vi "getRequirementsDoc.vi"(8 "error in (no error)":errorcluster, 11 "Path":path=path "C:/Users/rolalla/SE/Opps/2010/Harley Davidson/TestBuilder/Source/HD_TestBuilder(06152010)/Requirements Gateway 1.1/NIGEL Engine/Document/NIGEL Dynamic Test Requirements.doc") -> (0 "error out":errorcluster, 1 "Cancelled?":bool, 2 "Requirements":string[](array[string]), 3 "Req Doc Folder":path)   [LabVIEW 2011]
uses:
  Progress.vi
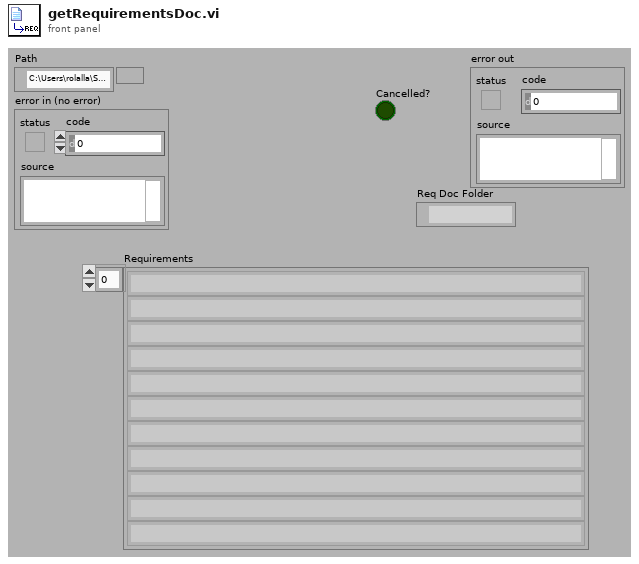
[diagram p1: front panel]
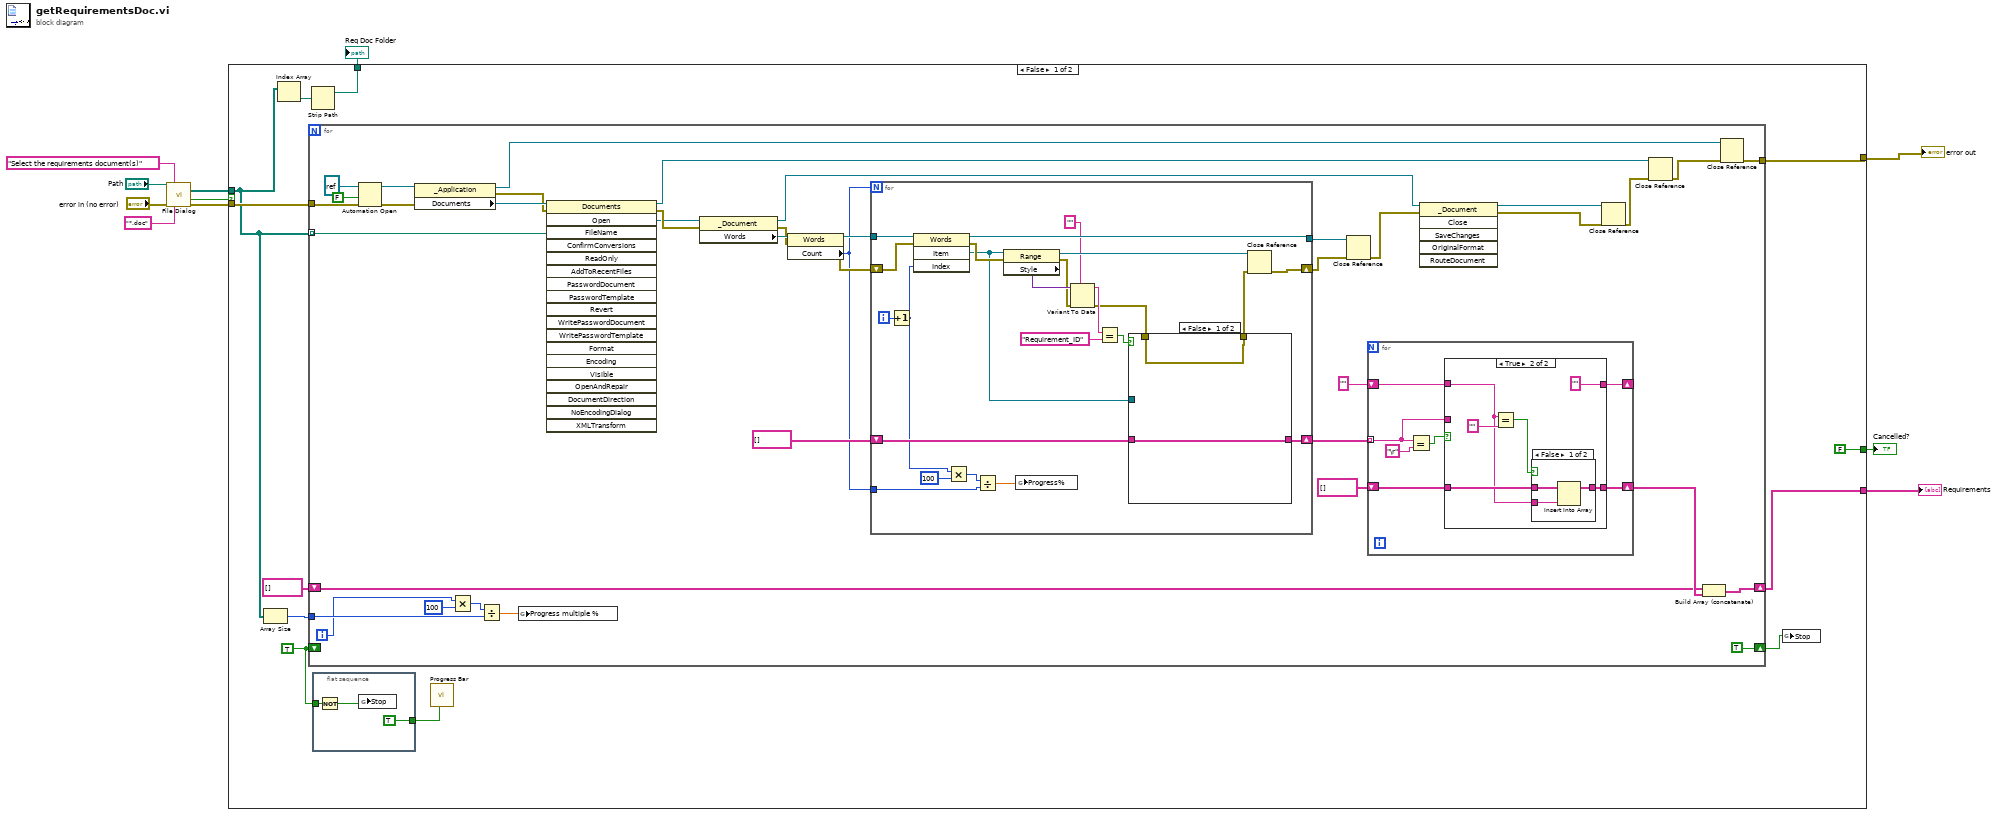
[diagram p0: block diagram]
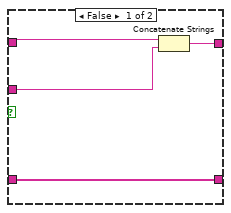
[diagram p2: hidden frame]
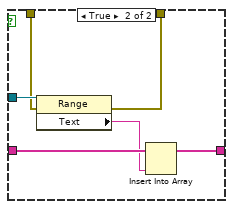
[diagram p4: hidden frame]
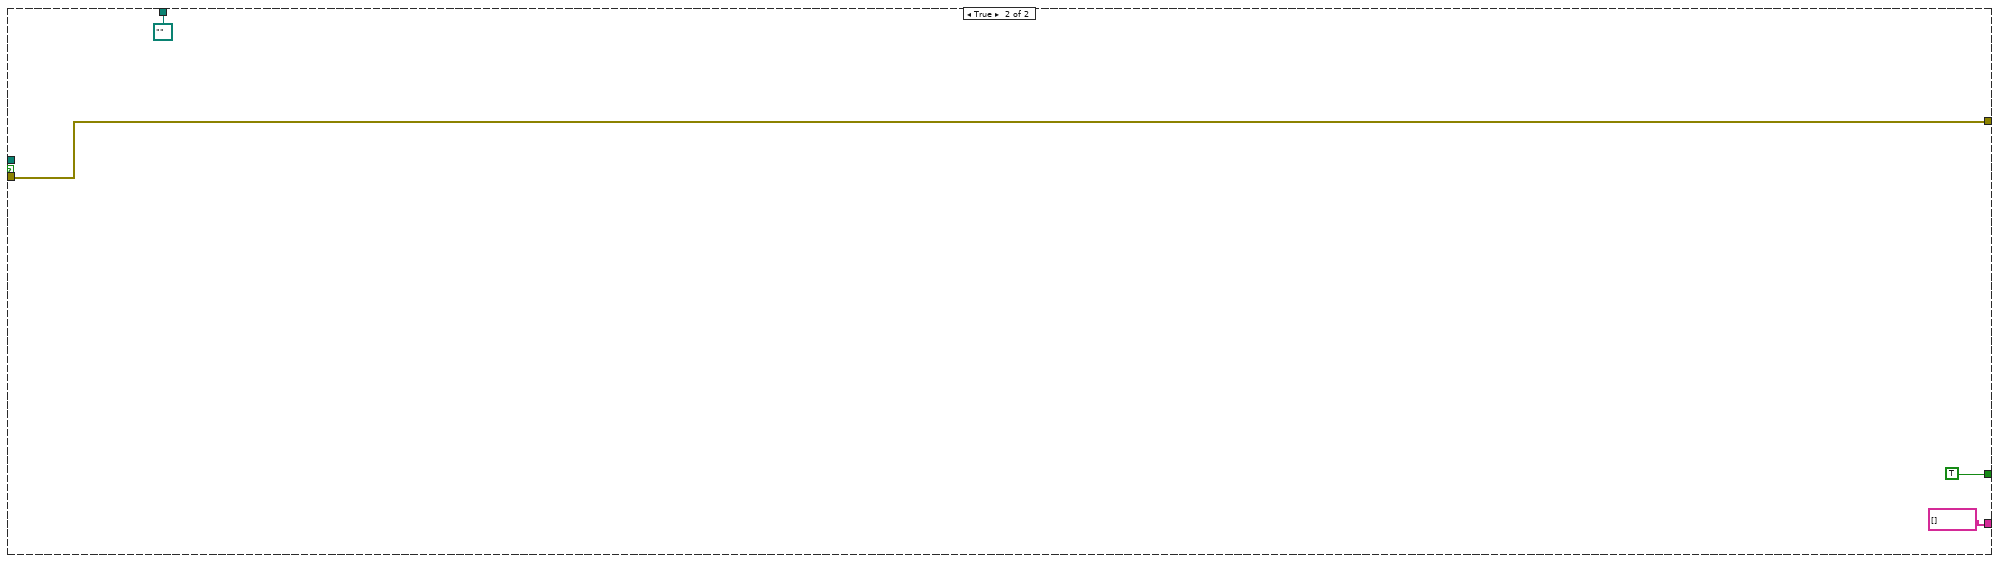
[diagram p5: hidden frame]
diagram:
  n1 = call "File Dialog"("start path"="Path", "prompt"="Select the requirements document(s)", "error in"="error in (no error)", "pattern (all files)"="*.doc") -> ("selected paths"=w4:path[], "cancelled"=w5:bool, "error out"=w6:errorcluster)  [unwired: 8 in, 1 out]
  n2 = case shown="False" w5 {
    tunnel: [w23 w121] -> w11
    tunnel: [w13 string[] []] -> w10
    tunnel: w6 -> [w22 w121]
    tunnel: w4 -> [w18 _]
    tunnel: [FALSE TRUE] -> w3
    tunnel: [w19 path "" ("stripped path")] -> w2
    frame False {
      w15 = TRUE
      n3 = Array Size(array=w18) -> (size(s)=w17:i32)
      n4 = Index Array(array=w18) -> (element=w20:path)  [unwired: 1 in]
      n5 = for {
        tunnel: [w61] -> w23
        tunnel: w22 -> [w57]
        tunnel: w18 -> [w56] mode=indexing
        tunnel: w17 -> [w33]
        shift-right: [TRUE] -> w16
        shift-left: w15 -> [_]
        shift-right: [w31] -> w13
        shift-left: string[] [] -> [w29]
        i -> [w32]
        n6 = Automation Open(error in (no error)=w57, Automation Refnum=refnum<k7> refnum ("Word._Application"), 9:FALSE ("open new instance (false)")) -> (Automation Refnum=w65:refnum<k7>, error out=w64:errorcluster)  [unwired: 1 in]
        n7 = property class="_Application"(reference=w65, error in=w64) -> (reference out=w60:refnum<k7>, error out=w58:errorcluster, "Documents"=w59:refnum<k7>)
        n8 = Multiply(x=w32, y=100) -> (x*y=w35:i32)
        n9 = Divide(x=w35, y=w33) -> (x/y=w27:dbl)
        n10 = global write "Progress.vi" "Progress multiple %"(w27) -> ()
        n11 = invoke class="Documents" method="Open"(reference=w59, error in=w58, "FileName"=w56) -> (reference out=w53:refnum<k7>, error out=w43:errorcluster, "Open"=w42:refnum<k7>)  [unwired: 16 in, 16 out]
        n12 = property class="_Document"(reference=w42, error in=w43) -> (reference out=w44:refnum<k7>, error out=w45:errorcluster, "Words"=w46:refnum<k7>)
        n13 = property class="Words"(reference=w46, error in=w45) -> (reference out=w52:refnum<k7>, error out=w37:errorcluster, "Count"=w28:i32)
        n14 = for {
          N: w28 -> [_]
          tunnel: w52 -> [w109]
          tunnel: [w103] -> w51
          shift-right: [w104] -> w50
          shift-left: w37 -> [w107]
          shift-right: [w92] -> w40
          shift-left: string[] [] -> [w93]
          tunnel: w28 -> [w88]
          i -> [w108]
          n15 = Increment(x=w108) -> (x+1=w89:i32)
          n16 = invoke class="Words" method="Item"(reference=w109, error in=w107, "Index"=w89) -> (reference out=w103:refnum<k7>, error out=w106:errorcluster, "Item"=w96:refnum<k7>)  [unwired: 1 in, 1 out]
          n17 = Multiply(x=w89, y=100) -> (x*y=w90:i32)
          n18 = Divide(x=w90, y=w88) -> (x/y=w87:dbl)
          n19 = property class="Range"(reference=w96, error in=w106) -> (reference out=w105:refnum<k7>, error out=w101:errorcluster, "Style"=w102:variant)
          n20 = global write "Progress.vi" "Progress%"(w87) -> ()
          n21 = Variant To Data(error in=w101, type="", Variant=w102) -> (data=w99:string, error out=w95:errorcluster)
          n22 = Equal?(x=w99, y="Requirement_ID") -> (x = y?=w97:bool)
          n23 = case shown="False" w97 {
            tunnel: w96 -> [_ w117]
            tunnel: w95 -> [w111 w116]
            tunnel: [w111 w115] -> w94
            tunnel: w93 -> [w110 w114]
            tunnel: [w110 w113] -> w92
            frame False {
            }
            frame True {
              n24 = property class="Range"(reference=w117, error in=w116) -> (error out=w115:errorcluster, "Text"=w112:string)  [unwired: 1 out]
              n25 = Insert Into Array(array=w114, new element=w112) -> (w113:string[])  [unwired: 1 in]
            }
          }
          n26 = Close Reference(reference=w105, error in (no error)=w94) -> (error out=w104:errorcluster)
        }
        n27 = Close Reference(reference=w51, error in (no error)=w50) -> (error out=w49:errorcluster)
        n28 = for {
          tunnel: w40 -> [w70] mode=indexing
          shift-right: [w68] -> _
          shift-left: "" -> [w69]
          shift-right: [w66] -> w30
          shift-left: string[] [] -> [w67]
          n29 = Equal?(x=w70, y="\r") -> (x = y?=w71:bool)
          n30 = case shown="True" w71 {
            tunnel: w70 -> [w75 _]
            tunnel: w69 -> [w76 w77]
            tunnel: [w74 ""] -> w68
            tunnel: w67 -> [w73 w82]
            tunnel: [w73 w81] -> w66
            frame False {
              n31 = Concatenate Strings(w76, w75) -> (w74:string)
            }
            frame True {
              n32 = Equal?(x=w77, y="") -> (x = y?=w78:bool)
              n33 = case shown="False" w78 {
                tunnel: w82 -> [w85 w86]
                tunnel: [w84 w86] -> w81
                tunnel: w77 -> [w83 _]
                frame False {
                  n34 = Insert Into Array(array=w85, new element=w83) -> (w84:string[])  [unwired: 1 in]
                }
                frame True {
                }
              }
            }
          }
        }
        n35 = invoke class="_Document" method="Close"(reference=w44, error in=w49) -> (reference out=w47:refnum<k7>, error out=w48:errorcluster)  [unwired: 4 in, 4 out]
        n36 = Close Reference(reference=w47, error in (no error)=w48) -> (error out=w54:errorcluster)
        n37 = Close Reference(reference=w53, error in (no error)=w54) -> (error out=w55:errorcluster)
        n38 = Build Array (concatenate)(w29, w30) -> (w31:string[])
        n39 = Close Reference(reference=w60, error in (no error)=w55) -> (error out=w61:errorcluster)
      }
      n40 = Strip Path(path=w20) -> (stripped path=w19:path)  [unwired: 1 out]
      n41 = flat-sequence {
        tunnel: w15 -> [w26]
        tunnel: [TRUE ("Multiple files?")] -> w12
        frame #0 {
          n42 = Not(x=w26) -> (.not. x?=w25:bool)
          n43 = global write "Progress.vi" "Stop"(w25) -> ()
        }
      }
      n44 = call "Progress Bar.vi"("Multiple files?"=w12) -> ()  [unwired: 11 in]
      n45 = global write "Progress.vi" "Stop"(w16) -> ()
    }
    frame True {
    }
  }
  "error out" <- w11
  "Requirements" <- w10
  "Cancelled?" <- w3
  "Req Doc Folder" <- w2
